vi "HP on far side.vi"(8 "LiftLocation":T1(ring)=enum."Cargo Zone 3", 9 "Z":dbl, 10 "Y":dbl, 11 "X":dbl) -> ()   [LabVIEW 2018]
uses:
  Robot Global Data.vi
  Hatch Panel Intake/Hatch Panel Intake Global.vi
panel:
  in  "Encoders":T2
  in  "PID Gains":T3={"X PID"={"proportional gain (Kc)"=0.02000000000000001, "integral time (Ti, min)"=0.0, "derivative time (Td, min)"=0.0}, "Y PID"={"proportional gain (Kc)"=0.02000000000000001, "integral time (Ti, min)"=0.0, "derivative time (Td, min)"=0.0}, "Z PID"={"proportional gain (Kc)"=0.02000000000000001, "integral time (Ti, min)"=0.0, "derivative time (Td, min)"=0.0}} {"Z PID"."derivative time (Td, min)" format="%.3f"; "Z PID"."integral time (Ti, min)" format="%.3f"; "Z PID"."proportional gain (Kc)" format="%.3f"; "Y PID"."derivative time (Td, min)" format="%.3f"; "Y PID"."integral time (Ti, min)" format="%.3f"; "Y PID"."proportional gain (Kc)" format="%.3f"; "X PID"."derivative time (Td, min)" format="%.3f"; "X PID"."integral time (Ti, min)" format="%.3f"; "X PID"."proportional gain (Kc)" format="%.3f"}
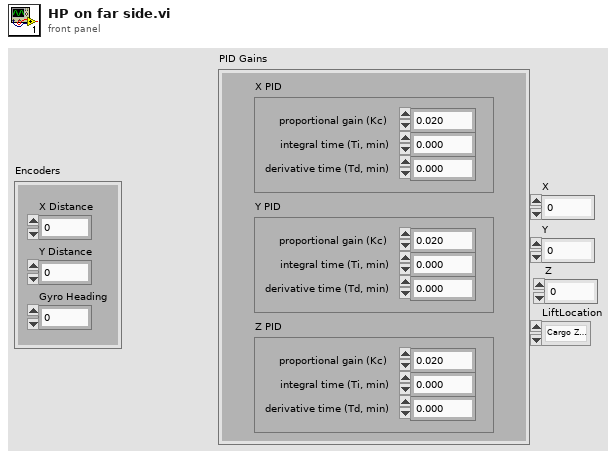
[diagram p1: front panel]
types:
  T1 = enum16{"N/A", "Hatch Panel Zone 1", "Hatch Panel Zone 2", "Hatch Panel Zone 3", "Cargo Zone 1", "Cargo Zone 2", "Cargo Zone 3"}
  T2 = cluster{"X Distance":dbl, "Y Distance":dbl, "Gyro Heading":dbl}
  T3 = cluster{"X PID":cluster{"proportional gain (Kc)":dbl, "integral time (Ti, min)":dbl, "derivative time (Td, min)":dbl}, "Y PID":cluster{"proportional gain (Kc)":dbl, "integral time (Ti, min)":dbl, "derivative time (Td, min)":dbl}, "Z PID":cluster{"proportional gain (Kc)":dbl, "integral time (Ti, min)":dbl, "derivative time (Td, min)":dbl}}
  T4 = cluster{"X Dist.":dbl, "Y Dist.":dbl, "Gyro":dbl}
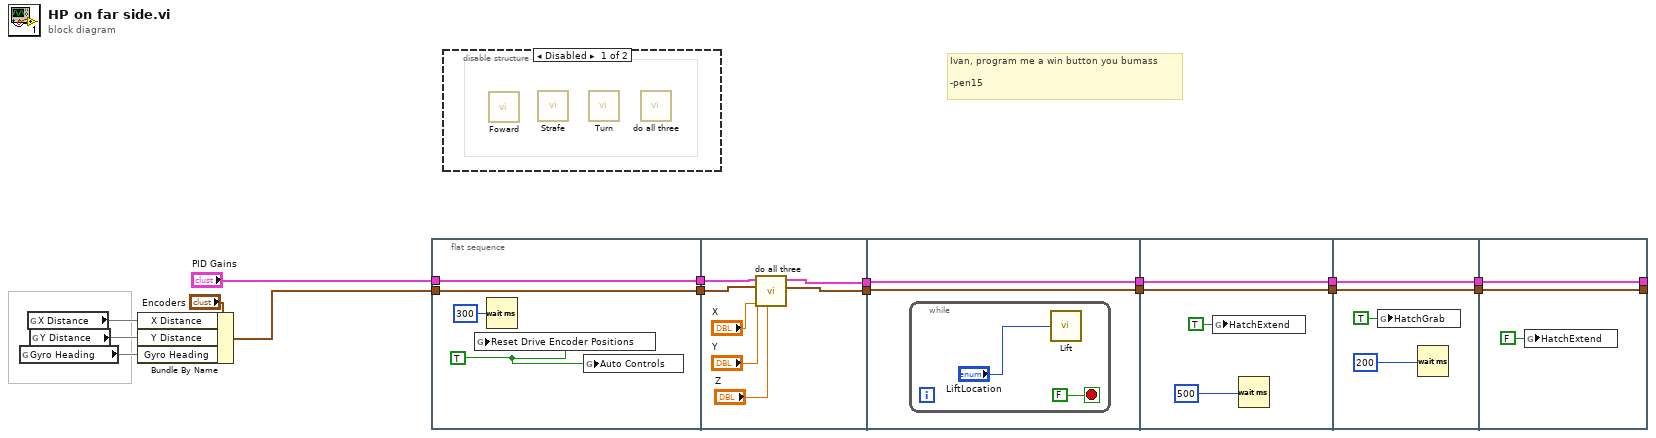
[diagram p0: block diagram]
diagram:
  # "Ivan, program me a win button you bumass\n\n-pen15"
  n1 = global read "Robot Global Data.vi" "Gyro Heading"() -> (w12)
  n2 = global read "Robot Global Data.vi" "X Distance"() -> (w10)
  n3 = global read "Robot Global Data.vi" "Y Distance"() -> (w11)
  n4 = Bundle By Name(cluster="Encoders", "X Distance"=w10, "Y Distance"=w11, "Gyro Heading"=w12) -> (w7:T2)
  n5 = flat-sequence {
    tunnel: [w18] -> w16
    tunnel: "PID Gains" -> [w18]
    tunnel: w7 -> [w17]
    tunnel: [w17] -> w15
    tunnel: w16 -> [w27]
    tunnel: w15 -> [w24]
    tunnel: [w26] -> w14
    tunnel: [w25] -> w13
    tunnel: [w28] -> w6
    tunnel: [w29] -> w5
    tunnel: w13 -> [w28]
    tunnel: w14 -> [w29]
    tunnel: w6 -> [w35]
    tunnel: w5 -> [w34]
    tunnel: [w35] -> w4
    tunnel: [w34] -> w3
    tunnel: w4 -> [w39]
    tunnel: w3 -> [w38]
    tunnel: [w39] -> w2
    tunnel: [w38] -> w1
    tunnel: [w41] -> _
    tunnel: [w42] -> _
    tunnel: w2 -> [w42]
    tunnel: w1 -> [w41]
    frame #0 {
      w20 = TRUE ("Auto Controls")
      n6 = global write "Robot Global Data.vi" "Reset Drive Encoder Positions"(w20) -> ()
      n7 = Wait (ms)(milliseconds to wait=u32 300) -> ()  [unwired: 1 out]
      n8 = global write "Robot Global Data.vi" "Auto Controls"(w20) -> ()
    }
    frame #1 {
      n9 = call "do all three.vi"("Gyro Target"="Z", "X Target"="X", "Y Target"="Y", "Encoders In"=w24, "PID Gains In"=w27) -> ("Encoders Out"=w25:T4, "PID Gains Out"=w26:T3)  [unwired: 5 in]
    }
    frame #2 {
      n10 = while {
        stop <- FALSE stop-if-true
        n11 = call "Lift.vi"("LiftLocation"="LiftLocation") -> ()
      }
    }
    frame #3 {
      n12 = global write "Hatch Panel Intake Global.vi" "HatchExtend"(TRUE ("HatchExtend")) -> ()
      n13 = Wait (ms)(milliseconds to wait=u32 500 ("millisecond timer value")) -> ()  [unwired: 1 out]
    }
    frame #4 {
      n14 = global write "Hatch Panel Intake Global.vi" "HatchGrab"(TRUE ("HatchGrab")) -> ()
      n15 = Wait (ms)(milliseconds to wait=u32 200 ("millisecond timer value")) -> ()  [unwired: 1 out]
    }
    frame #5 {
      n16 = global write "Hatch Panel Intake Global.vi" "HatchExtend"(FALSE ("HatchExtend")) -> ()
    }
  }
  n17 = disable-structure shown="Disabled" {
    frame Disabled {
      n18 = call "Foward.vi"() -> ()  [unwired: 9 in, 2 out]
      n19 = call "Strafe.vi"() -> ()  [unwired: 10 in, 2 out]
      n20 = call "Turn.vi"() -> ()  [unwired: 10 in, 2 out]
      n21 = call "do all three.vi"() -> ()  [unwired: 10 in, 2 out]
    }
    frame Enabled {
    }
  }
